vi "Write Controls to Config File.vi"(6 "Child?":bool, 7 "section":string, 8 "Error In":errorcluster, 9 "ParentName":string, 10 "Ctl Refnum":refnum<vi>, 11 "refnum":T1) -> (0 "Error Out":errorcluster, 3 "refnum out":T1)   [LabVIEW 2014]
uses:
  <vilib>/Utility/config.llb/Config Data RefNum.ctl
  Hardware/Table Stage/Controls/Translation Stage Cluster.ctl
  Controls/Translation Stage Types.ctl
  <vilib>/Utility/config.llb/Write Key (String).vi
  <vilib>/Utility/config.llb/Write Key (Path).vi
  <vilib>/Utility/config.llb/Write Key (Boolean).vi
  <vilib>/Utility/config.llb/Write Key (Double).vi
  <vilib>/Utility/config.llb/NI_LVConfig.lvlib
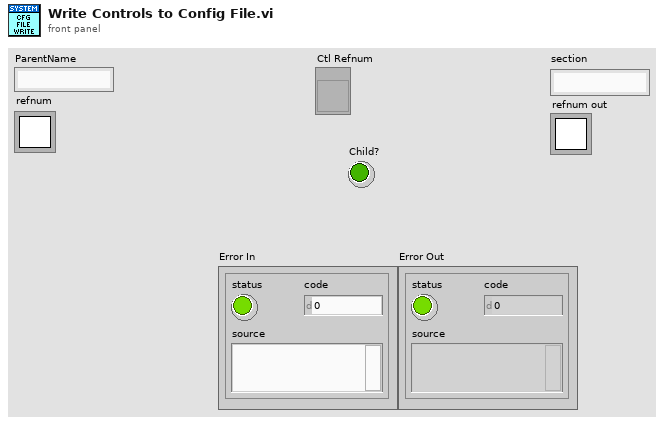
[diagram p1: front panel]
types:
  T1 = typedef "NI_LVConfig.lvlib/Config Data RefNum.ctl" = refnum<k1>
  T2 = typedef "Translation Stage Cluster.ctl" = cluster{"Position":dbl, "Is.Enabled?":bool, "Is.Connected?":bool, "Device SN":string, "AccelerationMaximum":dbl, "VelocityMaximum":dbl, "Acceleration":dbl, "Velocity":dbl, "waitTimeout (ms)":i32, "Model":T3, "Is.Homed?":bool}
  T3 = typedef "Translation Stage Types.ctl" = enum16{"None", "Thorlabs LTS", "Thorlabs MLJ"}
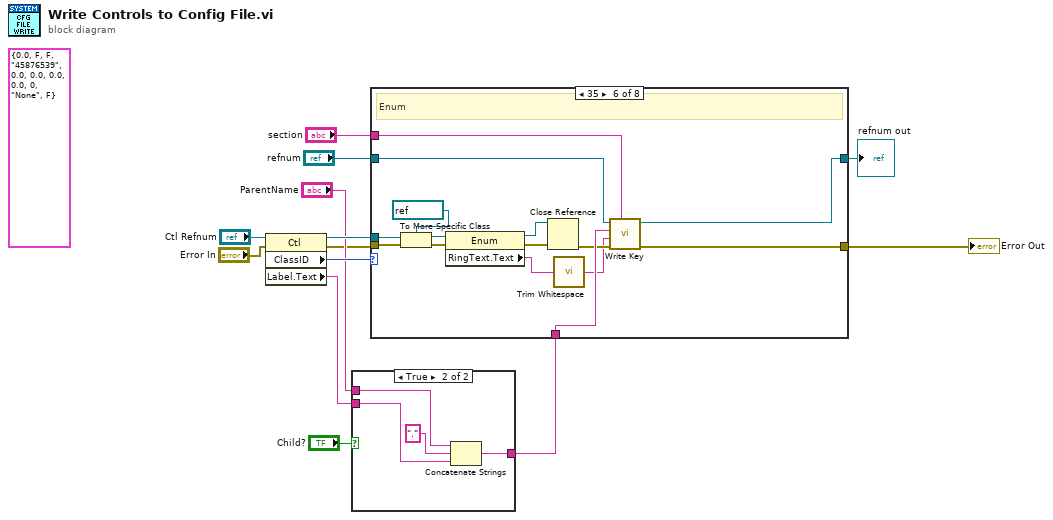
[diagram p0: block diagram]
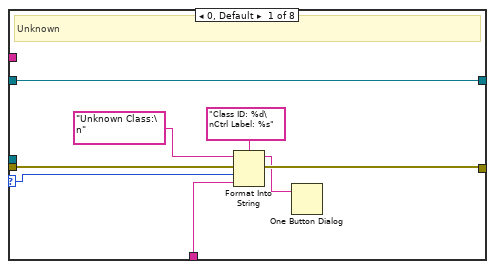
[diagram p3: hidden frame]
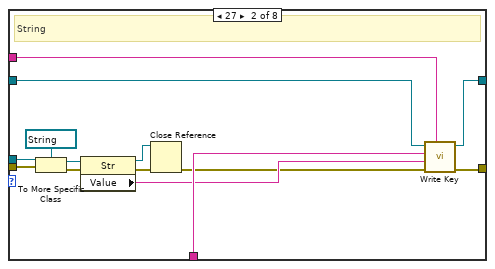
[diagram p4: hidden frame]
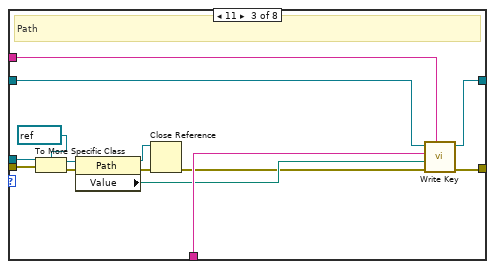
[diagram p5: hidden frame]
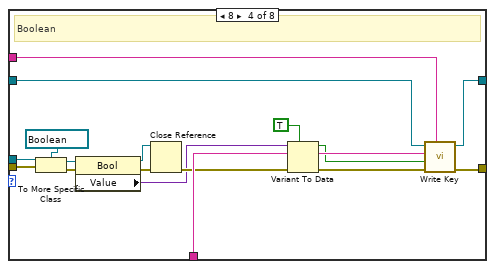
[diagram p6: hidden frame]
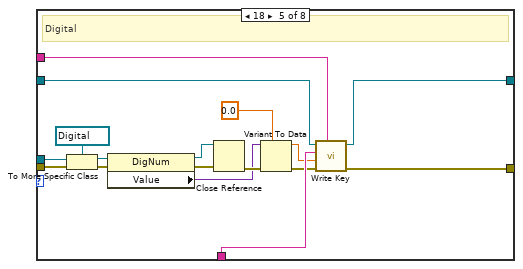
[diagram p7: hidden frame]
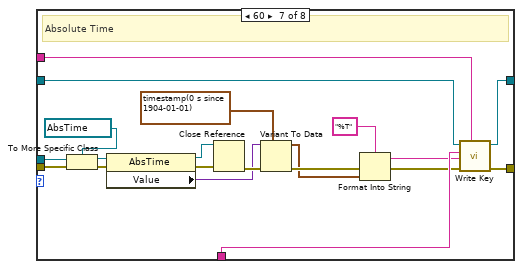
[diagram p8: hidden frame]
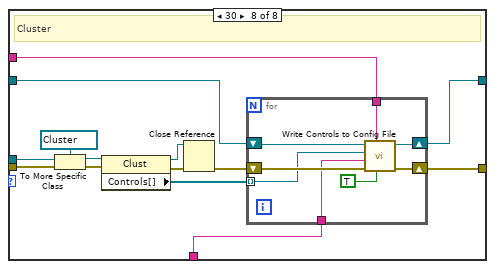
[diagram p9: hidden frame]
diagram:
  (unwired) T2 {"Position"=0.0, "Is.Enabled?"=FALSE, "Is.Connected?"=FALSE, "Device SN"="45876539", "AccelerationMaximum"=0.0, "VelocityMaximum"=0.0, "Acceleration"=0.0, "Velocity"=0.0, "waitTimeout (ms)"=0, "Model"=enum."None", "Is.Homed?"=FALSE} ("Control Param In")
  n1 = property class="Ctl"(reference="Ctl Refnum", error in="Error In") -> (reference out=w12:refnum<vi>, error out=w6:errorcluster, "ClassID"=w11:u32, "Label.Text"=w8:string)
  n2 = case shown="True" "Child?" {
    tunnel: "ParentName" -> [_ w18]
    tunnel: w8 -> [w14 w16]
    tunnel: [w14 w15] -> w3
    frame False {
    }
    frame True {
      n3 = Concatenate Strings(w18, ".", w16) -> (w15:string)
    }
  }
  n4 = case shown="35" w11 {
    selector: w11 -> [w23 _ _ _ _ _ _ _]
    tunnel: w6 -> [w21 w39 w54 w70 w88 w103 w123 w137]
    tunnel: w12 -> [_ w38 w53 w69 w87 w102 w122 w135]
    tunnel: [w20 w37 w52 w68 w76 w93 w112 w131] -> w1
    tunnel: "section" -> [_ w36 w51 w67 w79 w96 w115 w128]
    tunnel: "refnum" -> [w26 w35 w50 w66 w78 w95 w114 w130]
    tunnel: [w26 w34 w49 w65 w77 w94 w113 w129] -> w2
    tunnel: w3 -> [w22 w32 w47 w63 w80 w97 w116 w127]
    frame 0, Default {
      # "Unknown"
      n5 = Format Into String(format string="Class ID: %d\nCtrl Label: %s", initial string="Unknown Class:\n" ("string"), error in=w21, w23, w22) -> (resulting string=w19:string, error out=w20:errorcluster)
      n6 = One Button Dialog(message=w19) -> ()  [unwired: 1 in, 1 out]
    }
    frame 27 {
      # "String"
      n7 = To More Specific Class(target class=refnum<vi> refnum ("AccelerationMaximum 2"), reference=w38, error in=w39) -> (specific class reference=w30:refnum<vi>, error out=w33:errorcluster)
      n8 = property class="Str"(reference=w30, error in=w33) -> (reference out=w27:refnum<vi>, error out=w31:errorcluster, "Value"=w29:string)
      n9 = Close Reference(reference=w27, error in (no error)=w31) -> (error out=w28:errorcluster)
      n10 = call-poly <vilib>:"Write Key.vi"("section"=w36, "error in (no error)"=w28, "value"=w29, "key"=w32, "refnum"=w35) -> ("error out"=w37:errorcluster, "refnum out"=w34:T1)  [unwired: 4 in, 1 out]
    }
    frame 11 {
      # "Path"
      n11 = To More Specific Class(target class=refnum<vi> refnum ("Path"), reference=w53, error in=w54) -> (specific class reference=w45:refnum<vi>, error out=w48:errorcluster)
      n12 = property class="Path"(reference=w45, error in=w48) -> (reference out=w42:refnum<vi>, error out=w46:errorcluster, "Value"=w44:path)
      n13 = Close Reference(reference=w42, error in (no error)=w46) -> (error out=w43:errorcluster)
      n14 = call-poly <vilib>:"Write Key.vi"("section"=w51, "error in (no error)"=w43, "value"=w44, "key"=w47, "refnum"=w50) -> ("error out"=w52:errorcluster, "refnum out"=w49:T1)  [unwired: 4 in, 1 out]
    }
    frame 8 {
      # "Boolean"
      n15 = To More Specific Class(target class=refnum<vi> refnum ("AccelerationMaximum 2"), reference=w69, error in=w70) -> (specific class reference=w61:refnum<vi>, error out=w64:errorcluster)
      n16 = property class="Bool"(reference=w61, error in=w64) -> (reference out=w59:refnum<vi>, error out=w62:errorcluster, "Value"=w57:variant)
      n17 = Close Reference(reference=w59, error in (no error)=w62) -> (error out=w60:errorcluster)
      n18 = Variant To Data(error in=w60, type=TRUE, Variant=w57) -> (data=w55:bool, error out=w58:errorcluster)
      n19 = call-poly <vilib>:"Write Key.vi"("section"=w67, "error in (no error)"=w58, "value"=w55, "key"=w63, "refnum"=w66) -> ("error out"=w68:errorcluster, "refnum out"=w65:T1)  [unwired: 4 in, 1 out]
    }
    frame 18 {
      # "Digital"
      n20 = To More Specific Class(target class=refnum<vi> refnum ("AccelerationMaximum 2"), reference=w87, error in=w88) -> (specific class reference=w84:refnum<vi>, error out=w85:errorcluster)
      n21 = property class="DigNum"(reference=w84, error in=w85) -> (reference out=w82:refnum<vi>, error out=w83:errorcluster, "Value"=w74:variant)
      n22 = Close Reference(reference=w82, error in (no error)=w83) -> (error out=w81:errorcluster)
      n23 = Variant To Data(error in=w81, type=0.0, Variant=w74) -> (data=w72:dbl, error out=w75:errorcluster)
      n24 = call-poly <vilib>:"Write Key.vi"("section"=w79, "error in (no error)"=w75, "value"=w72, "key"=w80, "refnum"=w78) -> ("error out"=w76:errorcluster, "refnum out"=w77:T1)  [unwired: 4 in, 1 out]
    }
    frame 35 {
      # "Enum"
      n25 = To More Specific Class(target class=refnum<vi> refnum ("Enum"), reference=w102, error in=w103) -> (specific class reference=w100:refnum<vi>, error out=w101:errorcluster)
      n26 = property class="Enum"(reference=w100, error in=w101) -> (reference out=w98:refnum<vi>, error out=w99:errorcluster, "RingText.Text"=w90:string)
      n27 = Close Reference(reference=w98, error in (no error)=w99) -> (error out=w91:errorcluster)
      n28 = call <vilib>:"Trim Whitespace.vi"("string"=w90) -> ("trimmed string"=w89:string)  [unwired: 1 in]
      n29 = call-poly <vilib>:"Write Key.vi"("section"=w96, "error in (no error)"=w91, "value"=w89, "key"=w97, "refnum"=w95) -> ("error out"=w93:errorcluster, "refnum out"=w94:T1)  [unwired: 4 in, 1 out]
    }
    frame 60 {
      # "Absolute Time"
      n30 = To More Specific Class(target class=refnum<vi> refnum ("AccelerationMaximum 2"), reference=w122, error in=w123) -> (specific class reference=w120:refnum<vi>, error out=w121:errorcluster)
      n31 = property class="AbsTime"(reference=w120, error in=w121) -> (reference out=w118:refnum<vi>, error out=w119:errorcluster, "Value"=w110:variant)
      n32 = Close Reference(reference=w118, error in (no error)=w119) -> (error out=w117:errorcluster)
      n33 = Variant To Data(error in=w117, type=timestamp(0 s since 1904-01-01), Variant=w110) -> (data=w104:timestamp, error out=w111:errorcluster)
      n34 = Format Into String(format string="%T", error in=w111, w104) -> (resulting string=w108:string, error out=w109:errorcluster)  [unwired: 1 in]
      n35 = call-poly <vilib>:"Write Key.vi"("section"=w115, "error in (no error)"=w109, "value"=w108, "key"=w116, "refnum"=w114) -> ("error out"=w112:errorcluster, "refnum out"=w113:T1)  [unwired: 4 in, 1 out]
    }
    frame 30 {
      # "Cluster"
      n36 = To More Specific Class(target class=refnum<vi> refnum ("Cluster Ref In"), reference=w135, error in=w137) -> (specific class reference=w133:refnum<vi>, error out=w134:errorcluster)
      n37 = property class="Clust"(reference=w133, error in=w134) -> (reference out=w125:refnum<vi>, error out=w132:errorcluster, "Controls[]"=w124:refnum<vi>[])
      n38 = Close Reference(reference=w125, error in (no error)=w132) -> (error out=w126:errorcluster)
      n39 = for {
        tunnel: w128 -> [w141]
        tunnel: w127 -> [w140]
        shift-right: [w144] -> w131
        shift-left: w126 -> [w145]
        shift-right: [w142] -> w129
        shift-left: w130 -> [w143]
        tunnel: w124 -> [w138] mode=indexing
        n40 = call "Write Controls to Config File.vi"("Child?"=TRUE, "section"=w141, "Error In"=w145, "ParentName"=w140, "Ctl Refnum"=w138, "refnum"=w143) -> ("Error Out"=w144:errorcluster, "refnum out"=w142:T1)  [unwired: 4 in]
      }
    }
  }
  "Error Out" <- w1
  "refnum out" <- w2
